vi "Preset SCREEN query.vi"(8 "error in (no error)":errorcluster, 11 "VISA resource in":refnum<visa-resource-name>) -> (0 "error out":errorcluster, 2 "Result":string, 3 "VISA resource out":refnum<visa-resource-name>)   [LabVIEW 2025, in "Chroma 19572.lvlib"]
doc: "This VI writes to the instrument the SCREEN state."
uses:
  <instrlib>/Chroma 19572/Chroma 19572.lvlib
panel:
  # "PreSet SCREEN query"
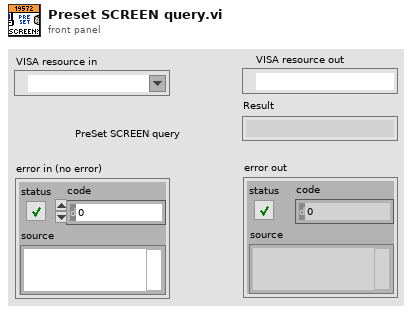
[diagram p1: front panel]
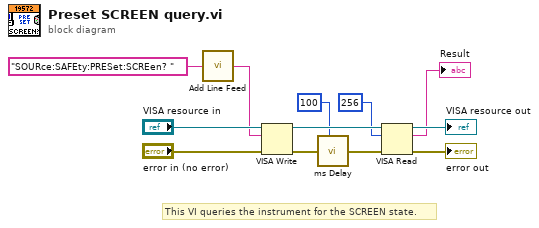
[diagram p0: block diagram]
diagram:
  # "This VI queries the instrument for the SCREEN state."
  n1 = call <instrlib>:"Add Line Feed.vi"("Command string"="SOURce:SAFEty:PRESet:SCREen? ") -> ("Concatenated string"=w4:string)  [unwired: 4 in]
  n2 = VISA Write(VISA resource name="VISA resource in", write buffer=w4, error in (no error)="error in (no error)") -> (VISA resource name out=w11:refnum<visa-resource-name>, error out=w10:errorcluster)  [unwired: 1 out]
  n3 = call <instrlib>:"ms Delay.vi"("miliseconds to wait"=u32 100 ("Time Delay ms"), "error in (no error)"=w10) -> ("error out"=w9:errorcluster)  [unwired: 6 in, 1 out]
  n4 = VISA Read(VISA resource name=w11, byte count=u32 256, error in (no error)=w9) -> (VISA resource name out=→"VISA resource out":refnum<visa-resource-name>, read buffer=→"Result":string, error out=→"error out":errorcluster)  [unwired: 1 out]
